vi "ClearSafeMode.vi"(7 "LabVIEW Web Service Request":refnum<class "Web Request.lvclass">) -> ()   [LabVIEW 2017]
uses:
  <vilib>/wsapi/Web Request.lvclass
  <vilib>/addons/Qbus/Qbus.lvclass
  <vilib>/addons/InsightCM/Devices/Shared/Common/Controller/Controller.lvlib
panel:
  out "error out":errorcluster
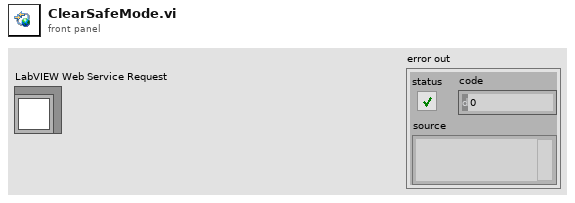
[diagram p1: front panel]
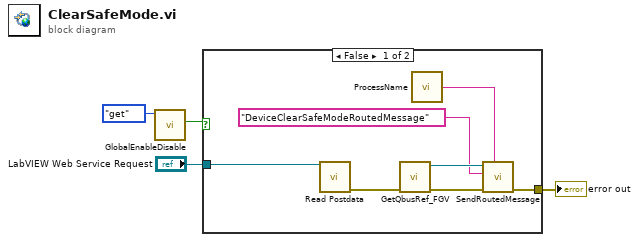
[diagram p0: block diagram]
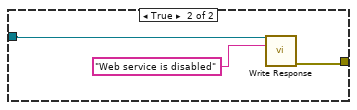
[diagram p2: hidden frame]
diagram:
  n1 = call "GlobalEnableDisable.vi"("action"=enum16{"init", "set", "get"}."get") -> ("DisableDeviceWebService"=w1:bool)  [unwired: 10 in]
  n2 = case shown="False" w1 {
    tunnel: "LabVIEW Web Service Request" -> [w11 w13]
    tunnel: [w5 w12] -> w3
    frame False {
      n3 = call <vilib>:"Read Postdata.vi"("LabVIEW Web Service Request"=w11) -> ("error out"=w10:errorcluster)  [unwired: 12 in, 2 out]
      n4 = call <vilib>:"GetQbusRef_FGV.vi"("error in (no error)"=w10) -> ("error out"=w6:errorcluster, "Qbus out"=w9:refnum<class "Qbus.lvclass">)  [unwired: 9 in]
      n5 = call <vilib>:"ProcessName.vi"() -> ("ProcessName"=w7:string)  [unwired: 5 in]
      n6 = call <vilib>:"SendRoutedMessage.vi"("listener process"=w7, "error in (no error)"=w6, "message name"="DeviceClearSafeModeRoutedMessage" ("scheduled exit reason"), "Qbus in"=w9) -> ("error in (no error)"=w5:errorcluster)  [unwired: 6 in, 1 out]
    }
    frame True {
      n7 = call <vilib>:"Write Response.vi"("LabVIEW Web Service Request"=w13, "response string"="Web service is disabled") -> ("error out"=w12:errorcluster)  [unwired: 12 in, 1 out]
    }
  }
  "error out" <- w3
